vi "Fetch&Process_Measurements_V4.vi"(0 "DCPowerInformation_byChannel":T1(array[cluster]), 5 "Initial Time":timestamp, 11 "error in (no error)":errorcluster) -> (2 "Current Reading too High?":bool[](array[boolean]), 3 "Latest Time":timestamp, 4 "Data As dbl Array":dbl[][][](array[numeric]), 6 "Channel Number Array":string[](array[string]), 8 "Current Waveform Array":waveform(dbl)[](array[waveform]), 10 "Voltage Waveform Array":waveform(dbl)[](array[waveform]), 14 "TimeStamp Array":timestamp[](array[timestamp]), 15 "error out":errorcluster)   [LabVIEW 2019]
uses:
  <vilib>/Analysis/1siggen.llb/Ramp Pattern by Delta.vi
  <vilib>/Analysis/NI_AALBase.lvlib
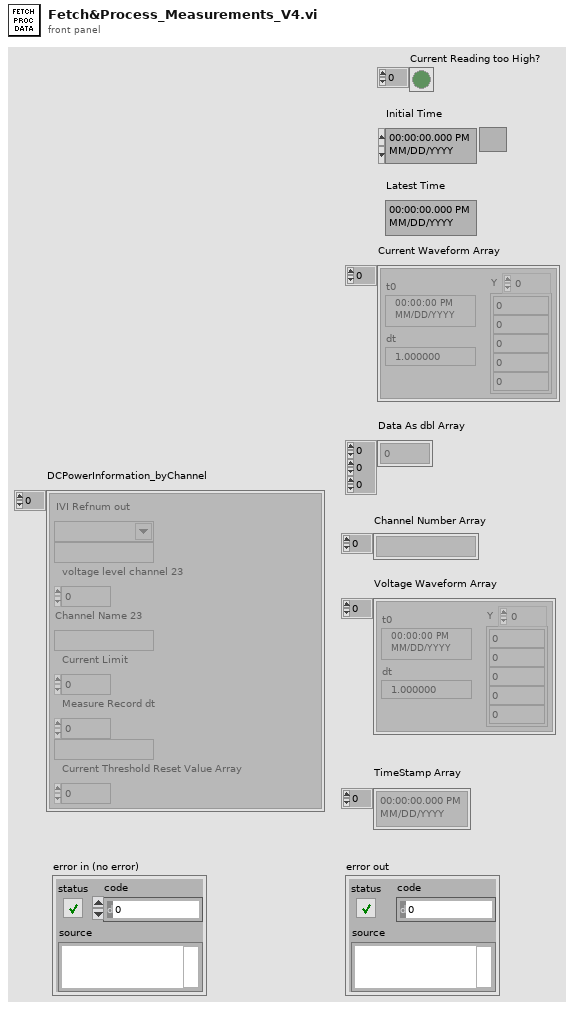
[diagram p1: front panel]
types:
  T1 = cluster{"IVI Refnum out":refnum<k15>, string, "voltage level channel 23":dbl, "Channel Name 23":string, "Current Limit":dbl, "Measure Record dt":dbl, string, "Current Threshold Reset Value Array":dbl}[]
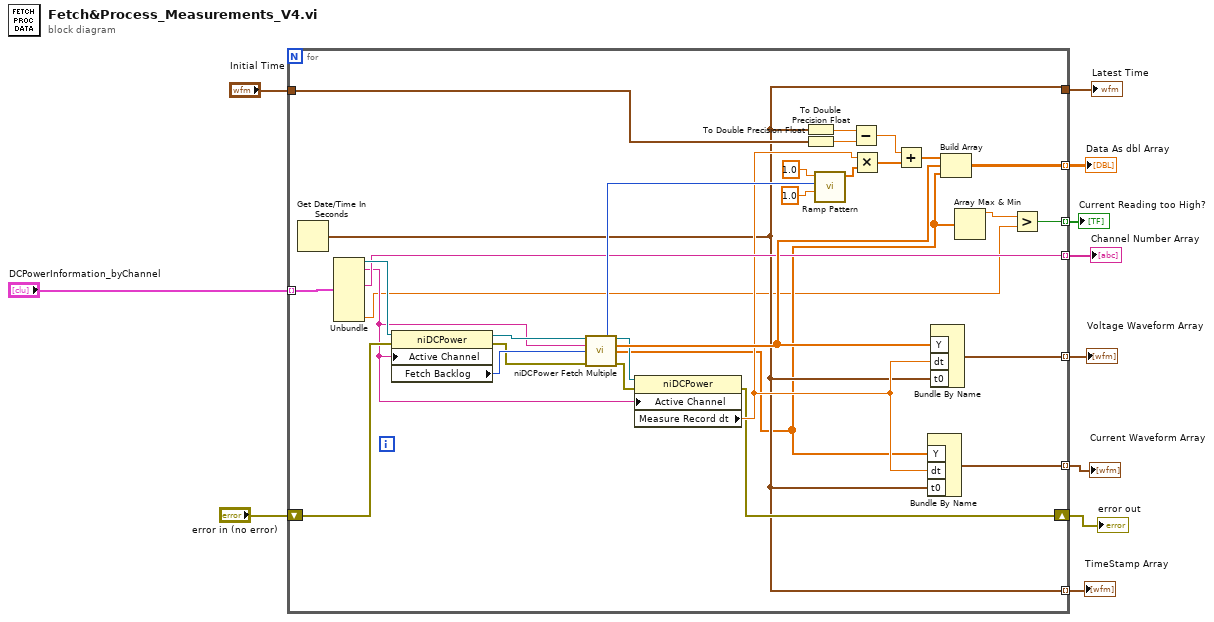
[diagram p0: block diagram]
diagram:
  n1 = for {
    tunnel: "DCPowerInformation_byChannel" -> [w20] mode=indexing
    tunnel: [w37] -> w7 mode=indexing
    tunnel: [w36] -> w8 mode=indexing
    shift-right: [w17] -> w6
    shift-left: "error in (no error)" -> [w41]
    tunnel: "Initial Time" -> [w25]
    tunnel: [w24] -> w10 mode=indexing
    tunnel: [w23] -> w11 mode=indexing
    tunnel: [w16] -> w4
    tunnel: [w16] -> w3 mode=indexing
    tunnel: [w12] -> w1 mode=indexing
    n2 = Get Date/Time In Seconds() -> (seconds since 1Jan1904=w16:timestamp)
    n3 = Unbundle(w20) -> ("IVI Refnum out"=w40:refnum<k15>, w18:string, "Channel Name 23"=w23:string, "Current Threshold Reset Value Array"=w13:dbl)  [unwired: 4 out]
    n4 = property class="niDCPower"(reference=w40, error in=w41, "Active Channel"=w18) -> (reference out=w39:refnum<k15>, error out=w38:errorcluster, "Fetch Backlog"=w42:i32)
    n5 = call <instrlib>:"niDCPower Fetch Multiple.vi"("instrument handle"=w39, "channel name"=w18, "count (1)"=w42, "error in (no error)"=w38) -> ("actual count"=w26:i32, "instrument handle out"=w22:refnum<k15>, "voltage measurements"=w27:dbl[], "current measurements"=w15:dbl[], "error out"=w21:errorcluster)  [unwired: 6 in, 1 out]
    n6 = property class="niDCPower"(reference=w22, error in=w21, "Active Channel"=w18) -> (error out=w17:errorcluster, "Measure Record dt"=w19:dbl)  [unwired: 1 out]
    n7 = To Double Precision Float(number=w16) -> (double precision float=w33:dbl)
    n8 = To Double Precision Float(number=w25) -> (double precision float=w32:dbl)
    n9 = call-poly <vilib>:"Ramp Pattern.vi"("start"=1.0, "end"=w26, "delta"=1.0) -> ("Ramp Pattern"=w29:dbl[])  [unwired: 6 in, 2 out]
    n10 = Subtract(x=w33, y=w32) -> (x-y=w30:dbl)
    n11 = Multiply(x=w19, y=w29) -> (x*y=w28:dbl[])
    n12 = Add(x=w30, y=w28) -> (x+y=w35:dbl[])
    n13 = Bundle By Name("Y"=w15, "dt"=w19, "t0"=w16) -> (w36:waveform(dbl))  [unwired: 1 out]
    n14 = Bundle By Name("Y"=w27, "dt"=w19, "t0"=w16) -> (w37:waveform(dbl))  [unwired: 1 out]
    n15 = Build Array(w35, w27, w15) -> (w24:dbl[][])
    n16 = Array Max & Min(array=w15) -> (max value=w14:dbl)  [unwired: 3 out]
    n17 = Greater?(x=w14, y=w13) -> (0:w12:bool)
  }
  "Channel Number Array" <- w11
  "Data As dbl Array" <- w10
  "Current Waveform Array" <- w8
  "Voltage Waveform Array" <- w7
  "error out" <- w6
  "Latest Time" <- w4
  "TimeStamp Array" <- w3
  "Current Reading too High?" <- w1
